vi "Load 1D String Array from File.vi"(7 "Remove empty strings?(T)":bool=TRUE, 8 "error in (no error)":errorcluster, 11 "File name":string) -> (0 "error out":errorcluster, 3 "Loaded 1D String Array":string[](array[string]))   [LabVIEW 2019, in "Project.Dependencies Finder.lvlib"]
uses:
  Project.Dependencies Finder.lvlib
  60fb194c-e5b2-41e8-b9b0-bb09cff871db.vi
  <vilib>/Utility/file.llb/Read Delimited Spreadsheet (string).vi
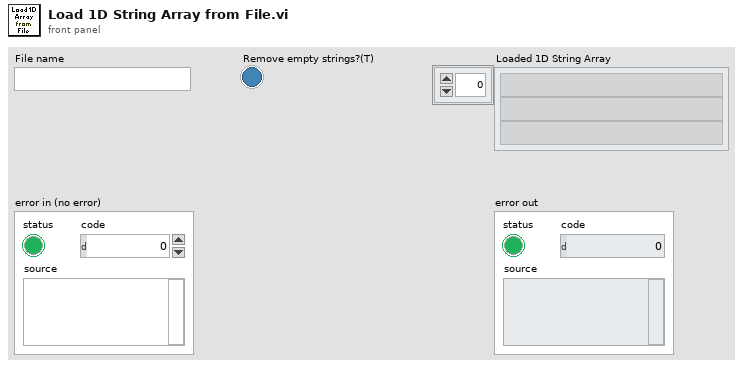
[diagram p1: front panel]
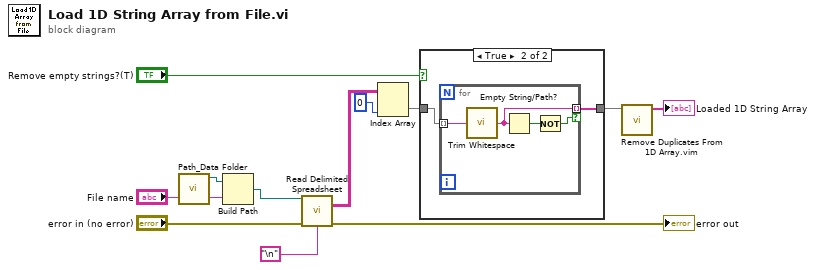
[diagram p0: block diagram]
diagram:
  n1 = call "Path_Data Folder.vi"() -> ("Data Folder Path"=w1:path)  [unwired: 11 in]
  n2 = Build Path(base path=w1, name or relative path="File name") -> (appended path=w4:path)
  n3 = call-poly <vilib>:"Read Delimited Spreadsheet.vi"("file path (dialog if empty)"=w4, "error in (no error)"="error in (no error)", "delimiter (\\t)"="\n") -> ("all rows"=w5:string[][], "error out"=→"error out":errorcluster)  [unwired: 7 in, 4 out]
  n4 = Index Array(array=w5, index (col)=0 ("disabled index (col)")) -> (element=w10:string[])  [unwired: 1 in]
  n5 = case shown="True" "Remove empty strings?(T)" {
    tunnel: [w13 w15] -> w11
    tunnel: w10 -> [w13 w14]
    frame False {
    }
    frame True {
      n6 = for {
        tunnel: w14 -> [w19] mode=indexing
        tunnel: [w17] -> w15 mode=indexing if=w16
        n7 = call <vilib>:"Trim Whitespace.vi"("string"=w19) -> ("trimmed string"=w17:string)  [unwired: 1 in]
        n8 = Empty String/Path?(string/path=w17) -> (empty?=w18:bool)
        n9 = Not(x=w18) -> (.not. x?=w16:bool)
      }
    }
  }
  n10 = call "Remove Duplicates From 1D Array.vim"("array"=w11) -> ("array with duplicates removed"=→"Loaded 1D String Array":string[])  [unwired: 10 in]
